vi "Do_channel_maths.vi"(4 "Output Index":i32, 5 "Channel Values In":string[][](array[string]), 6 "Channel Names":string[](array[string]), 7 "Maths Equation":string) -> (0 "Error String":string, 1 "Channel Values Out":string[][](array[string]), 3 "Results":dbl[](array[numeric]) format="%0.2f")   [LabVIEW 2016]
uses:
  Data_plotting_vis/Results_plotter_Global.vi
  <vilib>/gmath/NI_Gmath.lvlib
panel:
  out "Generic Equation":string
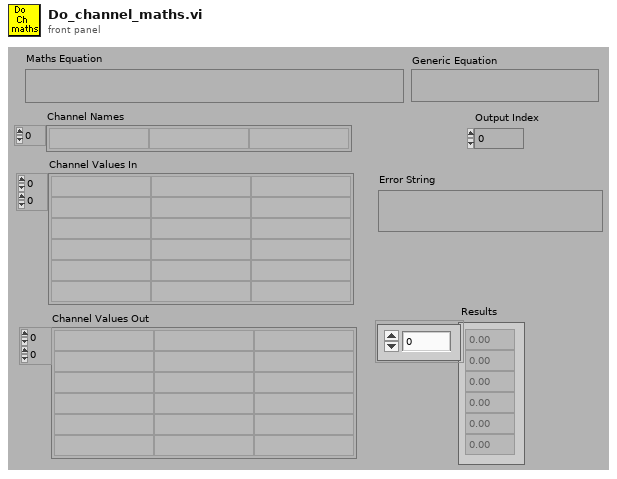
[diagram p1: front panel]
types:
  T1 = cluster{"Tables":i32[][], "Y Values":dbl[], "Variables input decode":i32[], i32[]}[]
  T2 = cluster{"Y Values":dbl[][], "Tables":i32[][][], "Variables input decode":i32[], "Variables output decode":i32[]}
  T3 = cluster{"Tables":i32[][], "Y Values":dbl[], "Variables input decode":i32[], i32[]}
  T4 = typedef "LVDateTimeRec.ctl" = cluster{"fractional second":dbl, "second":i32, "minute":i32, "hour":i32, "day of month":i32, "month":i32, "year":i32, "day of week":i32, "day of year":i32, "DST":i32}
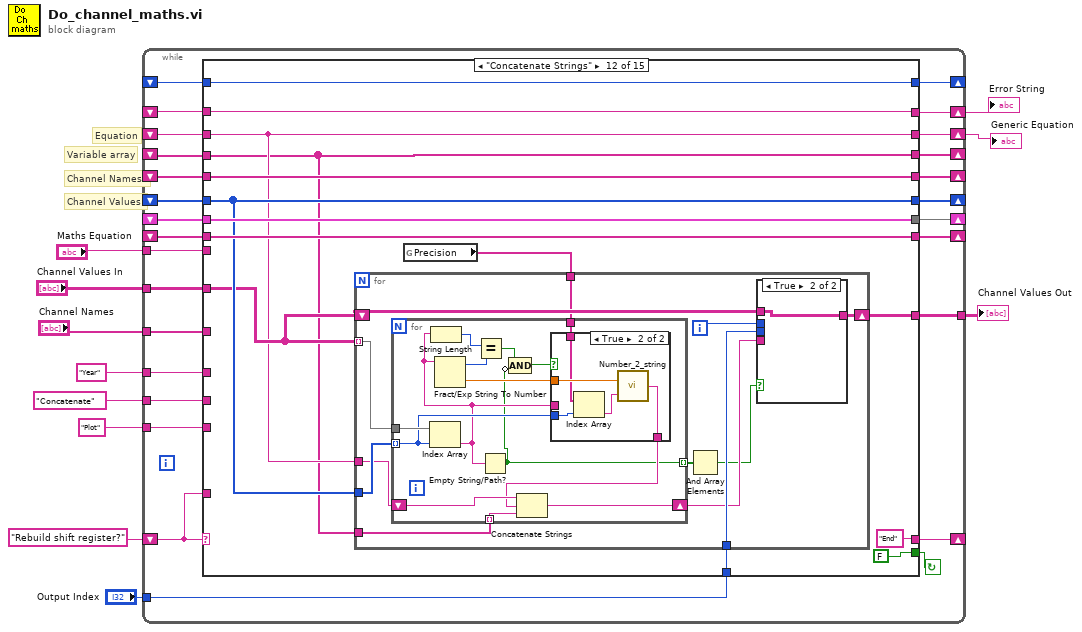
[diagram p0: block diagram]
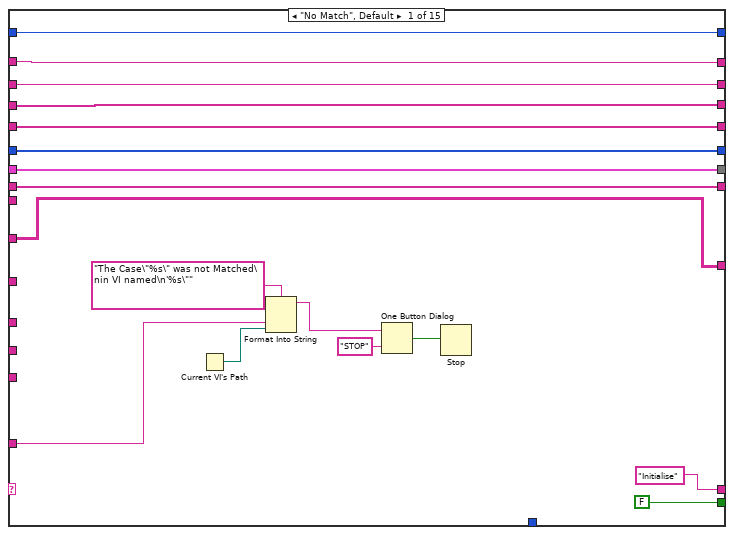
[diagram p2: hidden frame]
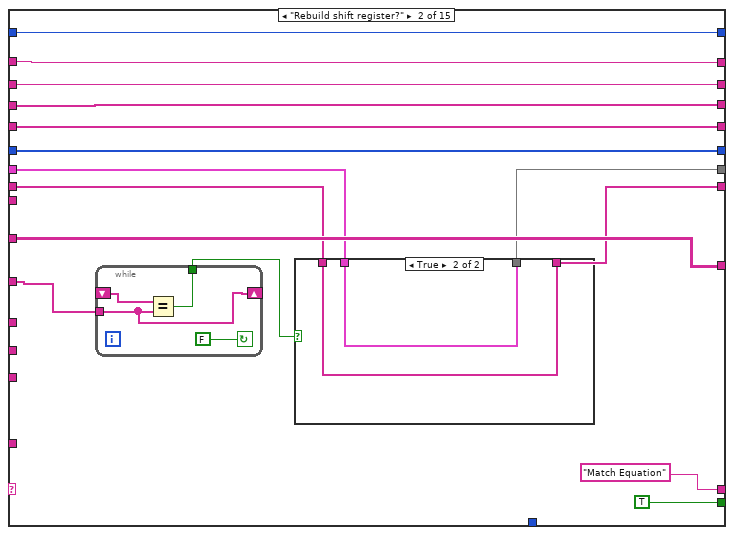
[diagram p3: hidden frame]
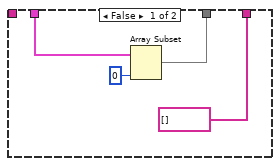
[diagram p4: hidden frame]
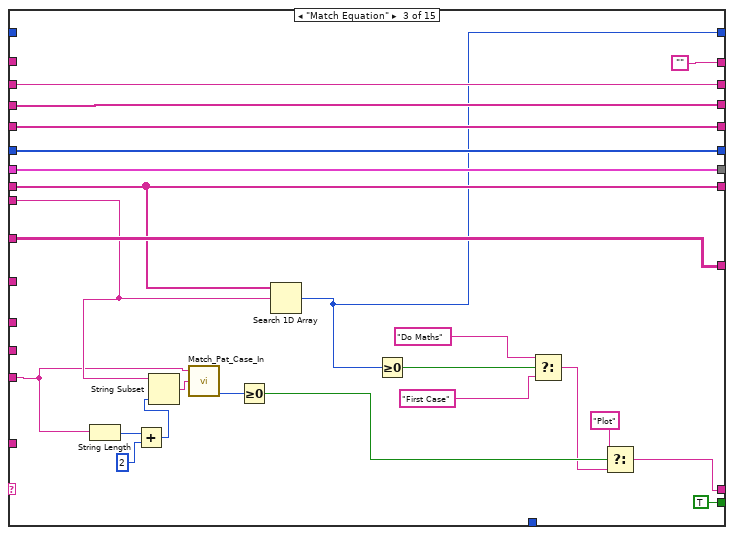
[diagram p5: hidden frame]
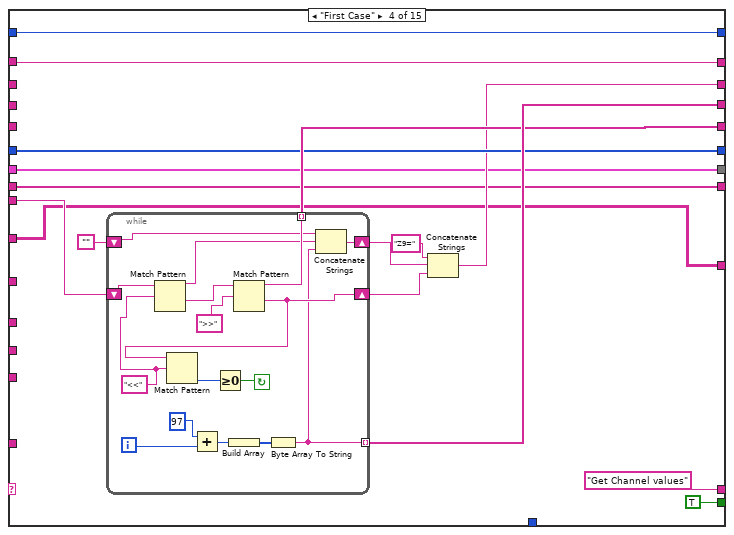
[diagram p6: hidden frame]
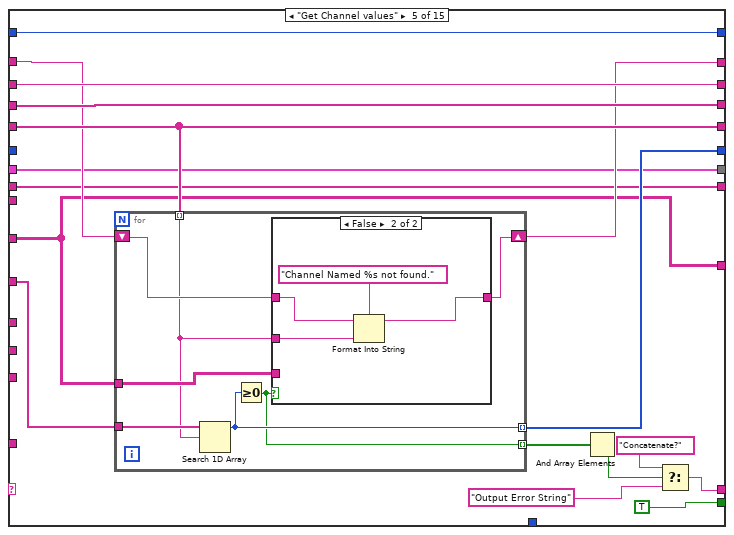
[diagram p7: hidden frame]
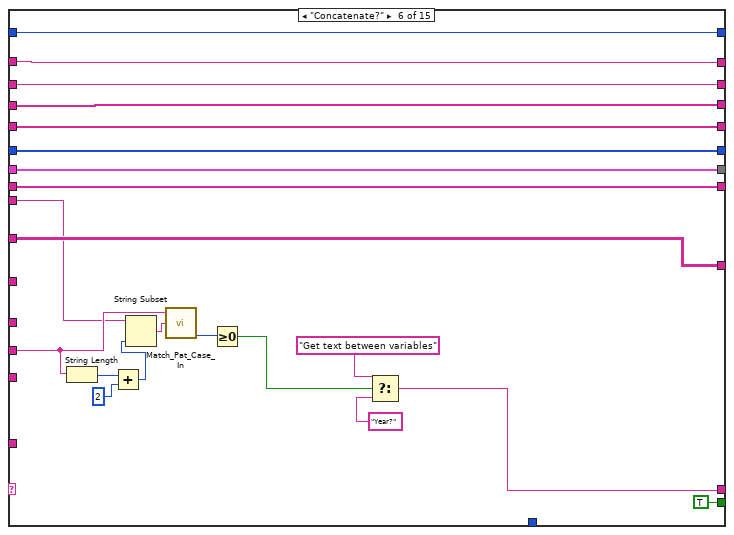
[diagram p9: hidden frame]
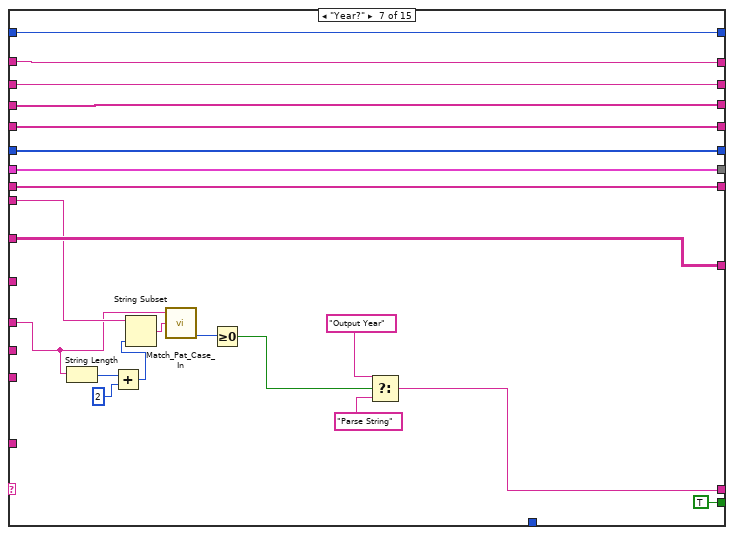
[diagram p10: hidden frame]
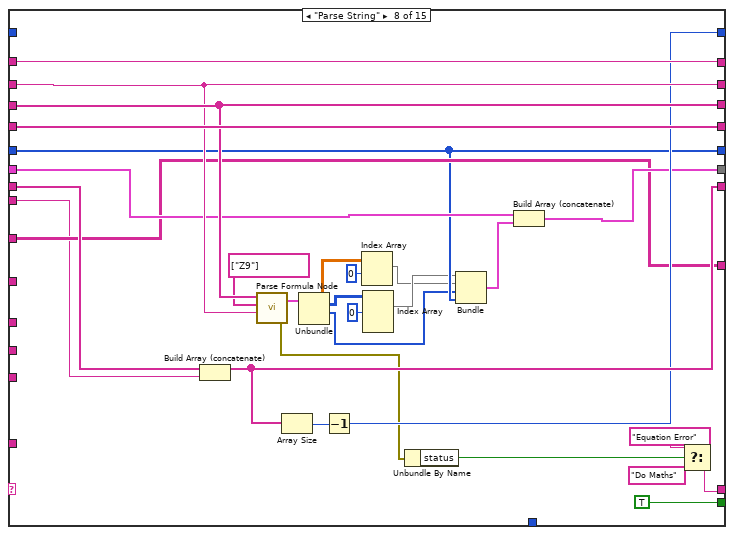
[diagram p11: hidden frame]
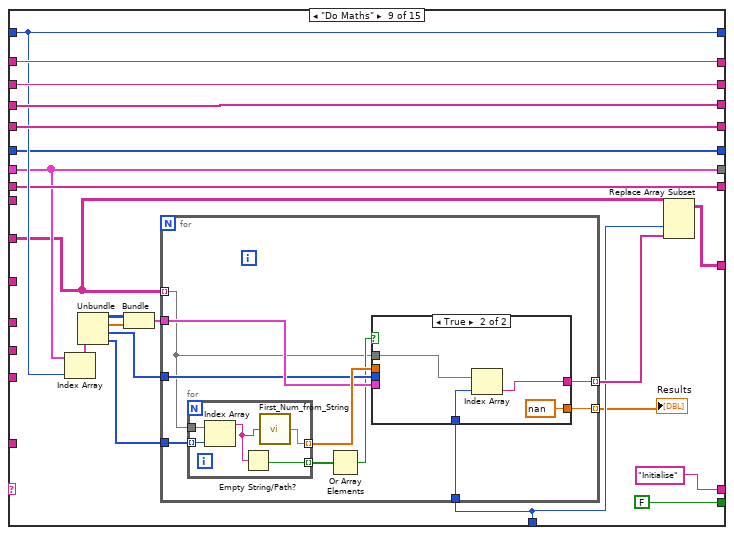
[diagram p12: hidden frame]
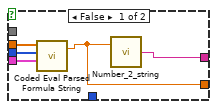
[diagram p13: hidden frame]
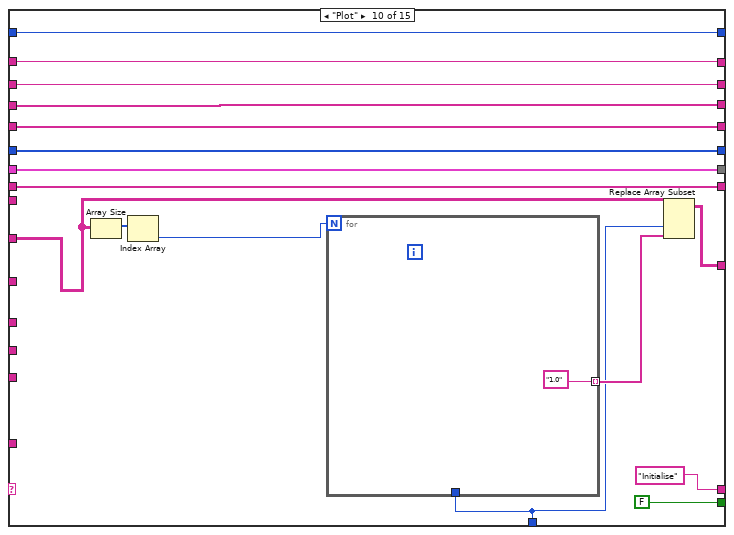
[diagram p14: hidden frame]
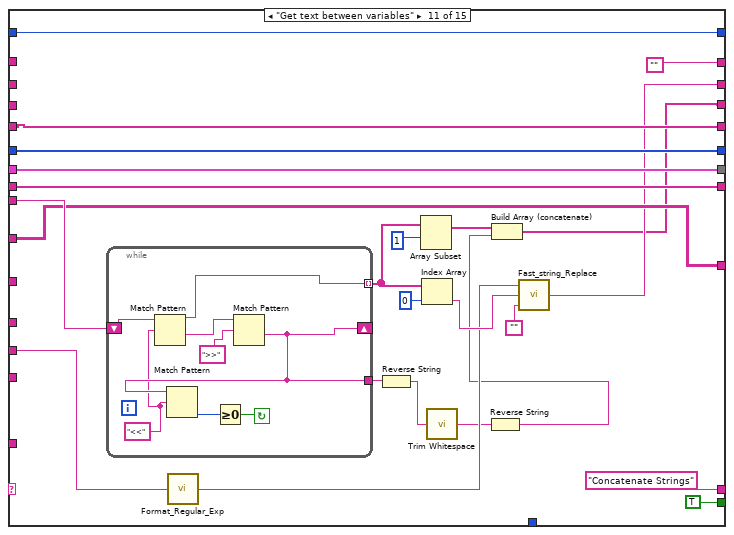
[diagram p15: hidden frame]
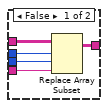
[diagram p16: hidden frame]
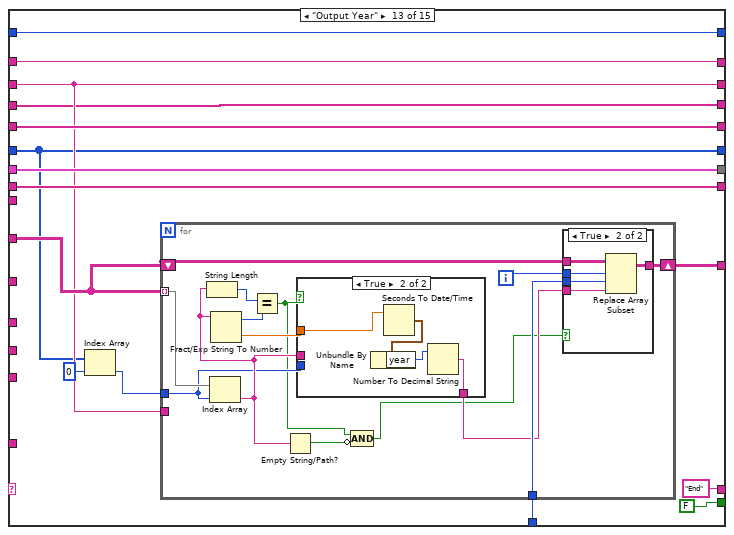
[diagram p18: hidden frame]
diagram:
  # "Channel Names"
  # "Variable array"
  # "Channel Values"
  # "Equation"
  n1 = while {
    tunnel: [w15] -> w5
    tunnel: "Output Index" -> [w16]
    shift-left: _ -> [w17]
    shift-right: [w18] -> _
    shift-left: _ -> [w21]
    shift-right: [w20] -> _
    shift-left: _ -> [w19]
    shift-right: [w22] -> _
    tunnel: "Channel Values In" -> [w23]
    tunnel: "Channel Names" -> [w24]
    tunnel: "Maths Equation" -> [w25]
    shift-left: _ -> [w27]
    shift-right: [w26] -> _
    shift-left: _ -> [w29]
    shift-right: [w28] -> _
    shift-left: _ -> [w31]
    shift-right: [w30] -> _
    shift-left: _ -> [w33]
    shift-right: [w32] -> w7
    shift-left: _ -> [w35]
    shift-right: [w34] -> w8
    shift-left: "Rebuild shift register?" -> [w36]
    shift-right: [w37] -> _
    tunnel: "Concatenate" ("regular expression") -> [w14]
    tunnel: "Plot" ("regular expression") -> [w13]
    tunnel: "Year" ("regular expression") -> [w12]
    stop <- w38 continue-if-true
    n2 = case shown="\"Concatenate Strings\"" w36 {
      tunnel: [FALSE TRUE TRUE TRUE TRUE TRUE TRUE TRUE FALSE FALSE TRUE FALSE FALSE TRUE FALSE] -> w38
      tunnel: ["Initialise" "Match Equation" w82 "Get Channel values" w138 w175 w196 w222 "Initialise" "Initialise" "Concatenate Strings" "End" "End" "Output Error String" "Initialise"] -> w37
      tunnel: w36 -> [w50 _ _ _ _ _ _ _ _ _ _ _ _ _ _]
      tunnel: w35 -> [w47 w68 _ w105 w146 w186 w207 w234 w254 w294 _ w341 w394 w424 w437]
      tunnel: [w47 w68 "" w105 w147 w186 w207 w234 w254 w294 "" w341 w394 w423 w437] -> w34
      tunnel: w33 -> [w46 w67 w104 _ w152 w185 w206 w230 w252 w292 _ w333 w387 w426 w447]
      tunnel: [w46 w67 w104 w110 w152 w185 w206 w230 w252 w292 w308 w333 w387 w426 w447] -> w32
      tunnel: w31 -> [w45 w66 w103 _ w151 w184 w205 w231 w253 w293 _ w332 w386 w433 w448]
      tunnel: [w45 w66 w103 w117 w151 w184 w205 w231 w253 w293 w303 w332 w386 w433 w448] -> w30
      tunnel: w29 -> [w44 w65 w102 _ w149 w183 w204 w235 w255 w295 w313 w342 w395 w434 w449]
      tunnel: [w44 w65 w102 w113 w149 w183 w204 w235 w255 w295 w313 w342 w395 w434 w449] -> w28
      tunnel: w27 -> [w43 w64 w101 w112 _ w182 w203 w221 w243 w288 w318 w337 w385 w429 w441]
      tunnel: [w43 w64 w101 w112 w148 w182 w203 w221 w243 w288 w318 w337 w385 w429 w441] -> w26
      tunnel: w25 -> [_ _ w88 w118 _ w168 w190 w208 _ _ w320 _ _ w425 _]
      tunnel: w24 -> [_ w61 _ _ w150 _ _ _ _ _ _ _ _ _ w439]
      tunnel: w23 -> [w39 w62 w99 w106 w142 w174 w195 w226 w241 w284 w314 w336 w390 w428 w440]
      tunnel: [w42 w59 w100 w109 w145 w181 w202 w227 w249 w289 w317 w338 w391 w430 w444] -> w22
      tunnel: w21 -> [w41 w57 w98 w108 w144 w180 w201 w233 w250 w290 w316 w339 w392 w431 w445]
      tunnel: [w41 w56 w98 w108 w144 w180 w201 w232 w250 w290 w316 w339 w392 w431 w445] -> w20
      tunnel: w19 -> [w42 w58 w100 w109 w145 w181 w202 w229 w249 w289 w317 w338 w391 w430 w444]
      tunnel: [w40 w63 w97 w107 w143 w179 w200 w228 w251 w291 w315 w340 w393 w432 w446] -> w18
      tunnel: w17 -> [w40 w63 _ w107 w143 w179 w200 _ w251 w291 w315 w340 w393 w432 w446]
      tunnel: w16 -> [_ _ _ _ _ _ _ _ w238 w285 _ w335 w389 _ w443]
      tunnel: [w39 w62 w99 w106 w142 w174 w195 w226 w240 w287 w314 w334 w388 w428 w442] -> w15
      tunnel: w14 -> [_ _ _ _ _ w173 _ _ _ _ w310 _ _ _ _]
      tunnel: w13 -> [_ _ w87 _ _ _ _ _ _ _ _ _ _ _ _]
      tunnel: w12 -> [_ _ _ _ _ _ w187 _ _ _ _ _ _ _ _]
      frame "No Match", Default {
        n3 = Current VI's Path() -> (path=w49:path)
        n4 = Format Into String(format string="The Case\"%s\" was not Matched\nin VI named\n'%s\"" ("Format String"), w50, w49) -> (resulting string=w53:string)  [unwired: 2 in, 1 out]
        n5 = One Button Dialog(message=w53, button name ("OK")="STOP") -> (true=w51:bool)
        n6 = Stop(stop? (T)=w51) -> ()
      }
      frame "Rebuild shift register?" {
        n7 = while {
          shift-right: [w79] -> _
          shift-left: _ -> [w80]
          tunnel: w61 -> [w79]
          tunnel: [w78] -> w60
          stop <- FALSE continue-if-true
          n8 = Equal?(x=w80, y=w79) -> (x = y?=w78:bool)
        }
        n9 = case shown="True" w60 {
          tunnel: [w72 w76] -> w59
          tunnel: w58 -> [w74 w76]
          tunnel: w57 -> [_ w75]
          tunnel: [string[] [] w75] -> w56
          frame False {
            n10 = Array Subset(array=w74, length=0) -> (w72:T1)  [unwired: 1 in]
          }
          frame True {
          }
        }
      }
      frame "Match Equation" {
        n11 = String Length(string=w87) -> (length=w89:i32)
        n12 = Add(x=w89, y=2) -> (x+y=w91:i32)
        n13 = String Subset(string=w88, length (rest)=w91) -> (substring=w92:string)  [unwired: 1 in]
        n14 = call "Match_Pat_Case_In.vi"("String to match"=w87, "String"=w92) -> ("offset past match"=w85:i32)  [unwired: 1 in, 3 out]
        n15 = Greater Or Equal To 0?(x=w85) -> (x >= 0?=w84:bool)
        n16 = Search 1D Array(1D array=w98, element=w88) -> (index of element=w97:i32)  [unwired: 1 out]
        n17 = Greater Or Equal To 0?(x=w97) -> (x >= 0?=w96:bool)
        n18 = Select(t="Do Maths", s=w96, f="First Case") -> (s? t:f=w83:string)
        n19 = Select(t="Plot", s=w84, f=w83) -> (s? t:f=w82:string)
      }
      frame "First Case" {
        n20 = while {
          shift-left: "" -> [w123]
          shift-right: [w124] -> w115
          tunnel: [w125] -> w117 mode=indexing
          tunnel: [w131] -> w113 mode=indexing
          shift-left: w118 -> [w136]
          shift-right: [w134] -> w114
          i -> [w127]
          stop <- w132 continue-if-true
          w122 = "<<" ("regular expression")
          n21 = Match Pattern(string=w136, regular expression=w122) -> (before substring=w126:string, after substring=w135:string)  [unwired: 3 out]
          n22 = Add(x=97, y=w127) -> (x+y=w129:i32)
          n23 = Build Array(w129) -> (w130:i32[])
          n24 = Match Pattern(string=w135, regular expression=">>") -> (before substring=w131:string, after substring=w134:string)  [unwired: 3 out]
          n25 = Match Pattern(string=w134, regular expression=w122) -> (offset past match=w133:i32)  [unwired: 4 out]
          n26 = Greater Or Equal To 0?(x=w133) -> (x >= 0?=w132:bool)
          n27 = Byte Array To String(unsigned byte array=w130) -> (string=w125:string)
          n28 = Concatenate Strings(w123, w126, w125) -> (w124:string)
        }
        n29 = Concatenate Strings("Z9=" ("Substring"), w115, w114) -> (w110:string)
      }
      frame "Get Channel values" {
        n30 = for {
          tunnel: w150 -> [w160]
          tunnel: w149 -> [w156] mode=indexing
          tunnel: w142 -> [w159]
          tunnel: [w155] -> w148 mode=indexing
          shift-right: [w157] -> w147
          shift-left: w146 -> [w158]
          tunnel: [w154] -> w141 mode=indexing
          n31 = Search 1D Array(1D array=w160, element=w156) -> (index of element=w155:i32)  [unwired: 1 out]
          n32 = Greater Or Equal To 0?(x=w155) -> (x >= 0?=w154:bool)
          n33 = case shown="False" w154 {
            tunnel: w159 -> [_ _]
            tunnel: w156 -> [_ w165]
            tunnel: w158 -> [w161 w163]
            tunnel: [w161 w162] -> w157
            frame True {
            }
            frame False {
              n34 = Format Into String(format string="Channel Named %s not found." ("Format String"), initial string=w163, w165) -> (resulting string=w162:string)  [unwired: 1 in, 1 out]
            }
          }
        }
        n35 = And Array Elements(Boolean array=w141) -> (logical AND=w140:bool)
        n36 = Select(t="Concatenate?", s=w140, f="Output Error String") -> (s? t:f=w138:string)
      }
      frame "Concatenate?" {
        n37 = String Length(string=w173) -> (length=w172:i32)
        n38 = Add(x=w172, y=2) -> (x+y=w170:i32)
        n39 = String Subset(string=w168, length (rest)=w170) -> (substring=w169:string)  [unwired: 1 in]
        n40 = call "Match_Pat_Case_In.vi"("String to match"=w173, "String"=w169) -> ("offset past match"=w178:i32)  [unwired: 1 in, 3 out]
        n41 = Greater Or Equal To 0?(x=w178) -> (x >= 0?=w167:bool)
        n42 = Select(t="Get text between variables" ("regular expression"), s=w167, f="Year?" ("regular expression")) -> (s? t:f=w175:string)
      }
      frame "Year?" {
        n43 = String Length(string=w187) -> (length=w194:i32)
        n44 = Add(x=w194, y=2) -> (x+y=w192:i32)
        n45 = String Subset(string=w190, length (rest)=w192) -> (substring=w191:string)  [unwired: 1 in]
        n46 = call "Match_Pat_Case_In.vi"("String to match"=w187, "String"=w191) -> ("offset past match"=w199:i32)  [unwired: 1 in, 3 out]
        n47 = Greater Or Equal To 0?(x=w199) -> (x >= 0?=w189:bool)
        n48 = Select(t="Output Year" ("regular expression"), s=w189, f="Parse String" ("regular expression")) -> (s? t:f=w196:string)
      }
      frame "Parse String" {
        n49 = Build Array (concatenate)(w233, w208) -> (w232:string[])
        n50 = call <vilib>:"Parse Formula Node.vi"("formula"=w230, "Variables Output"=string[] ["Z9"], "Variables Input"=w231) -> ("error out"=w209:errorcluster, "Parsed Formula Node"=w218:T2)  [unwired: 1 in]
        n51 = Array Size(array=w232) -> (size(s)=w219:i32)
        n52 = Unbundle(w218) -> ("Y Values"=w217:dbl[][], "Tables"=w214:i32[][][], "Variables input decode"=w211:i32[])  [unwired: 1 out]
        n53 = Decrement(x=w219) -> (x-1=w228:i32)
        n54 = Index Array(array=w217, index (row)=0 ("Index")) -> (element=w212:dbl[])  [unwired: 1 in]
        n55 = Index Array(array=w214, index (dim 0)=0 ("Index")) -> (element=w213:i32[][])  [unwired: 2 in]
        n56 = Unbundle By Name(w209) -> ("status"=w225:bool)
        n57 = Bundle("Tables"=w213, "Y Values"=w212, "Variables input decode"=w211, w221) -> (w210:T3)  [unwired: 1 out]
        n58 = Build Array (concatenate)(w229, w210) -> (w227:T1)
        n59 = Select(t="Equation Error", s=w225, f="Do Maths") -> (s? t:f=w222:string)
      }
      frame "Do Maths" {
        n60 = Index Array(array=w249, index=w251) -> (element=w248:T3)
        n61 = Unbundle(w248) -> ("Tables"=w247:i32[][], "Y Values"=w246:dbl[], "Variables input decode"=w244:i32[], w242:i32[])
        n62 = Bundle("Tables"=w247, "Y Values"=w246) -> (w245:cluster{"Tables":i32[][], "Y Values":dbl[]})  [unwired: 1 out]
        n63 = for {
          tunnel: w241 -> [w260] mode=indexing
          tunnel: w242 -> [w267]
          tunnel: w245 -> [w265]
          tunnel: w244 -> [w264]
          tunnel: [w261] -> w239 mode=indexing
          tunnel: w238 -> [w259]
          tunnel: [w258] -> w237 mode=indexing
          n64 = for {
            tunnel: w260 -> [w281]
            tunnel: w267 -> [w280] mode=indexing
            tunnel: [w277] -> w266 mode=indexing
            tunnel: [w279] -> w263 mode=indexing
            n65 = Index Array(array=w281, index=w280) -> (element=w278:string)
            n66 = Empty String/Path?(string/path=w278) -> (empty?=w279:bool)
            n67 = call "First_Num_from_String.vi"("string"=w278) -> ("number"=w277:dbl)
          }
          n68 = Or Array Elements(Boolean array=w263) -> (logical OR=w262:bool)
          n69 = case shown="True" w262 {
            tunnel: w266 -> [w272 _]
            tunnel: w265 -> [w271 _]
            tunnel: w264 -> [w270 _]
            tunnel: [w269 w274] -> w261
            tunnel: w260 -> [_ w276]
            tunnel: w259 -> [_ w275]
            tunnel: [w268 nan ("y value")] -> w258
            frame False {
              n70 = call <vilib>:"Coded Eval Parsed Formula String.vi"("Parsed Formula"=w271, "Variables"=w270, "X Values"=w272) -> ("y value"=w268:dbl)  [unwired: 1 in, 1 out]
              n71 = call "Number_2_string.vi"("number"=w268) -> ("String"=w269:string)  [unwired: 1 in]
            }
            frame True {
              n72 = Index Array(array=w276, index=w275) -> (element=w274:string)
            }
          }
        }
        "Results" <- w237
        n73 = Replace Array Subset(array=w241, new element=w239, index (col)=w238) -> (w240:string[][])  [unwired: 1 in]
      }
      frame "Plot" {
        n74 = Array Size(array=w284) -> (size(s)=w283:i32[])
        n75 = Index Array(array=w283) -> (element=w282:i32)  [unwired: 1 in]
        n76 = for {
          N: w282 -> [_]
          tunnel: ["1.0"] -> w286 mode=indexing
          tunnel: w285 -> [_]
        }
        n77 = Replace Array Subset(array=w284, new element=w286, index (col)=w285) -> (w287:string[][])  [unwired: 1 in]
      }
      frame "Get text between variables" {
        n78 = while {
          shift-left: w320 -> [w330]
          shift-right: [w325] -> _
          tunnel: [w326] -> w306 mode=indexing
          tunnel: [w325] -> w302
          stop <- w327 continue-if-true
          w324 = "<<" ("regular expression")
          n79 = Match Pattern(string=w330, regular expression=w324) -> (before substring=w326:string, after substring=w329:string)  [unwired: 3 out]
          n80 = Match Pattern(string=w329, regular expression=">>") -> (after substring=w325:string)  [unwired: 4 out]
          n81 = Match Pattern(string=w325, regular expression=w324) -> (offset past match=w328:i32)  [unwired: 4 out]
          n82 = Greater Or Equal To 0?(x=w328) -> (x >= 0?=w327:bool)
        }
        n83 = call "Format_Regular_Exp.vi"("Regular expression"=w310) -> ("Case Insensitive for html"=w309:string)
        n84 = Reverse String(1:w302) -> (0:w301:string)
        n85 = Array Subset(array=w306, index=1) -> (w305:string[])  [unwired: 1 in]
        n86 = Index Array(array=w306, index=0) -> (element=w311:string)
        n87 = call <vilib>:"Trim Whitespace.vi"("string"=w301) -> ("trimmed string"=w300:string)  [unwired: 1 in]
        n88 = Reverse String(1:w300) -> (0:w299:string)
        n89 = Build Array (concatenate)(w305, w299) -> (w303:string[])
        n90 = call "Fast_string_Replace.vi"("Replace match with:"="", "Input String"=w311, "regular expression"=w309) -> ("Output String"=w308:string)  [unwired: 2 out]
      }
      frame "Concatenate Strings" {
        n91 = global read "Results_plotter_Global.vi" "Precision"() -> (w331:string[])
        n92 = for {
          tunnel: w336 -> [w356] mode=indexing
          shift-right: [w353] -> w334
          shift-left: w336 -> [w354]
          tunnel: w337 -> [w355]
          tunnel: w335 -> [w351]
          tunnel: w333 -> [w350]
          tunnel: w332 -> [w349]
          tunnel: w331 -> [w348]
          i -> [w352]
          n93 = for {
            tunnel: w356 -> [w376]
            tunnel: w355 -> [w369] mode=indexing
            shift-right: [w367] -> w347
            shift-left: w350 -> [w375]
            tunnel: w349 -> [w374] mode=indexing
            tunnel: w348 -> [w368]
            tunnel: [w364] -> w346 mode=indexing
            n94 = Index Array(array=w376, index=w369) -> (element=w366:string)
            n95 = String Length(string=w366) -> (length=w373:i32)
            n96 = Fract/Exp String To Number(string=w366) -> (offset past number=w372:i32, number=w371:dbl)  [unwired: 3 out]
            n97 = Equal?(x=w373, y=w372) -> (x = y?=w365:bool)
            n98 = Empty String/Path?(string/path=w366) -> (empty?=w364:bool)
            n99 = Compound Arithmetic op=AND(w365, invert w364) -> (w363:bool)
            n100 = case shown="True" w363 {
              tunnel: w371 -> [_ w382]
              tunnel: [w377 w381] -> w370
              tunnel: w366 -> [w377 _]
              tunnel: w369 -> [_ w380]
              tunnel: w368 -> [_ w379]
              frame False {
              }
              frame True {
                n101 = Index Array(array=w379, index=w380) -> (element=w378:string)
                n102 = call "Number_2_string.vi"("precision"=w378, "number"=w382) -> ("String"=w381:string)
              }
            }
            n103 = Concatenate Strings(w375, w370, w374) -> (w367:string)
          }
          n104 = And Array Elements(Boolean array=w346) -> (logical AND=w345:bool)
          n105 = case shown="True" w345 {
            tunnel: w354 -> [w361 w362]
            tunnel: [w360 w362] -> w353
            tunnel: w352 -> [w359 _]
            tunnel: w351 -> [w358 _]
            tunnel: w347 -> [w357 _]
            frame False {
              n106 = Replace Array Subset(array=w361, new element=w357, index (row)=w359, index (col)=w358) -> (w360:string[][])
            }
            frame True {
            }
          }
        }
      }
      frame "Output Year" {
        n107 = Index Array(array=w385, index=0) -> (element=w383:i32)
        n108 = for {
          tunnel: w390 -> [w411] mode=indexing
          shift-right: [w409] -> w388
          shift-left: w390 -> [w410]
          tunnel: w389 -> [w407]
          tunnel: w387 -> [_]
          tunnel: w383 -> [w402]
          i -> [w408]
          n109 = Index Array(array=w411, index=w402) -> (element=w403:string)
          n110 = String Length(string=w403) -> (length=w406:i32)
          n111 = Fract/Exp String To Number(string=w403) -> (offset past number=w405:i32, number=w404:dbl)  [unwired: 3 out]
          n112 = Equal?(x=w406, y=w405) -> (x = y?=w399:bool)
          n113 = Empty String/Path?(string/path=w403) -> (empty?=w400:bool)
          n114 = case shown="True" w399 {
            tunnel: w404 -> [_ w416]
            tunnel: [w412 w413] -> w401
            tunnel: w403 -> [w412 _]
            tunnel: w402 -> [_ _]
            frame False {
            }
            frame True {
              n115 = Seconds To Date/Time(time stamp (now)=w416) -> (date time rec=w415:T4)  [unwired: 1 in]
              n116 = Unbundle By Name(w415) -> ("year"=w414:i32)
              n117 = Number To Decimal String(number=w414) -> (decimal integer string=w413:string)  [unwired: 1 in]
            }
          }
          n118 = Compound Arithmetic op=AND(w399, invert w400) -> (w398:bool)
          n119 = case shown="True" w398 {
            tunnel: w410 -> [w417 w422]
            tunnel: [w417 w421] -> w409
            tunnel: w408 -> [_ w420]
            tunnel: w407 -> [_ w419]
            tunnel: w401 -> [_ w418]
            frame False {
            }
            frame True {
              n120 = Replace Array Subset(array=w422, new element=w418, index (row)=w420, index (col)=w419) -> (w421:string[][])
            }
          }
        }
      }
      frame "Equation Error" {
        n121 = Format Into String(format string="There is an error in the Maths Equation %s. The full equation is %s", initial string=w424, w426, w425) -> (resulting string=w423:string)  [unwired: 1 in, 1 out]
      }
      frame "Output Error String" {
        n122 = Array Size(array=w439) -> (size(s)=w438:i32)
        n123 = for {
          N: w438 -> [_]
          shift-right: [w455] -> w442
          shift-left: w440 -> [w456]
          tunnel: w443 -> [w453]
          tunnel: w437 -> [w452]
          i -> [w454]
          n124 = Replace Array Subset(array=w456, new element=w452, index (row)=w454, index (col)=w453) -> (w455:string[][])
        }
      }
    }
  }
  "Error String" <- w8
  "Generic Equation" <- w7
  "Channel Values Out" <- w5
